vi "Send Save to TDMS.vi"(4 "Stop Time":dbl[unit]=0.1, 6 "Start Time":dbl[unit]=-0.1, 7 "Message Priority (Normal)":T1=enum."Normal", 8 "error in (no error)":errorcluster, 9 "Quench Channel":i32, 10 "Quench Start":dbl[unit], 11 "Message Enqueuer":refnum<class "Message Enqueuer.lvclass">) -> (0 "error out":errorcluster, 3 "Message Enqueuer out":refnum<class "Message Enqueuer.lvclass">)   [LabVIEW 2015, in "KIT-QA.lvlib" / "Save to TDMS Msg.lvclass"]
doc: "This VI sends the message to an actor."
uses:
  Save to TDMS Msg.lvclass
  <vilib>/ActorFramework/Message Enqueuer/Message Enqueuer.lvclass
  <vilib>/ActorFramework/Message Enqueuer/Message Priority.ctl
  Save to TDMS Msg.lvclass/Save to TDMS Msg.ctl
  <vilib>/ActorFramework/Message Enqueuer/Message Enqueuer.lvclass/Message Enqueuer.ctl
  <vilib>/ActorFramework/Message Priority Queue/Priority Enqueue.vi
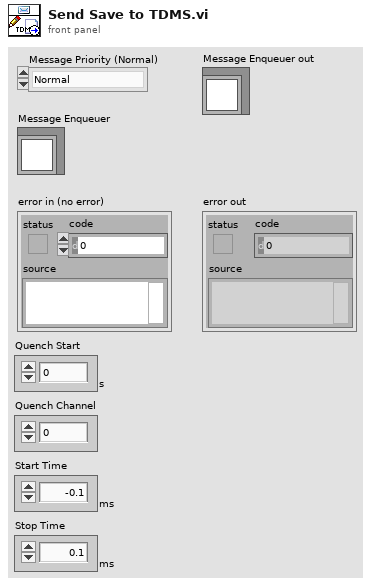
[diagram p1: front panel]
types:
  T1 = typedef "Actor Framework.lvlib/Message Enqueuer.lvclass/Message Priority.ctl" = enum16{"Low", "Normal", "High"}
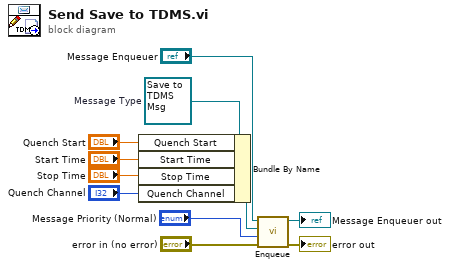
[diagram p0: block diagram]
diagram:
  w5 = refnum<class "Save to TDMS Msg.lvclass"> refnum  # Message Type
  n1 = Bundle By Name(cluster=w5, "Quench Start"="Quench Start", "Start Time"="Start Time", "Stop Time"="Stop Time", "Quench Channel"="Quench Channel") -> (w4:refnum<class "Save to TDMS Msg.lvclass">)
  n2 = call <vilib>:"Enqueue.vi"("error in (no error)"="error in (no error)", "Message Priority (Normal)"="Message Priority (Normal)", "Message"=w4, "Message Enqueuer in"="Message Enqueuer") -> ("error out"=→"error out":errorcluster, "Message Enqueuer out"=→"Message Enqueuer out":refnum<class "Message Enqueuer.lvclass">)  [unwired: 6 in]
